vi "Read Active Channels.vi"(8 "error in (no error)":errorcluster, 11 "Hardware Settings in":refnum<class "Hardware Settings.lvclass">) -> (0 "error out":errorcluster, 2 "Active Channels":refnum<class "Generic Hardware.lvclass">[](array[class]), 3 "Hardware Settings out":refnum<class "Hardware Settings.lvclass">)   [LabVIEW 2017, in "Hardware Settings.lvclass"]
uses:
  Hardware Settings.lvclass
  Hardware Types/Generic/Generic Hardware.lvclass
  Hardware Settings.lvclass/Hardware Settings.ctl
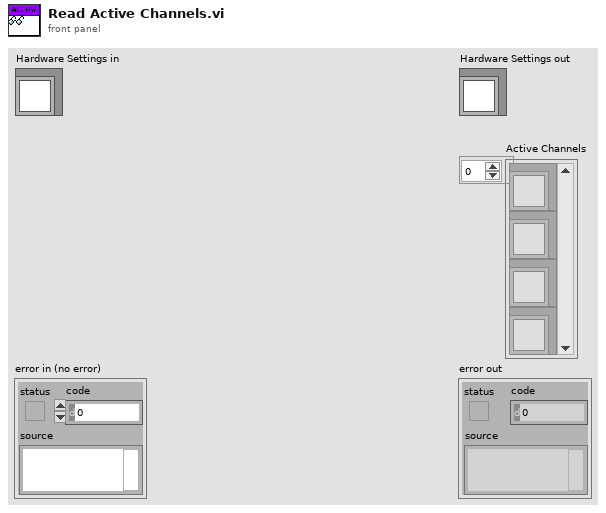
[diagram p1: front panel]
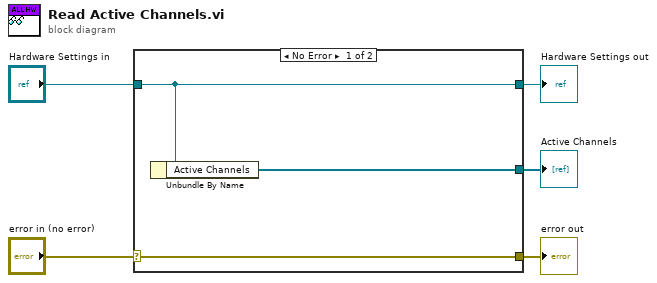
[diagram p0: block diagram]
diagram:
  n1 = case shown="No Error" "error in (no error)" {
    selector: "error in (no error)" -> [w8 w9]
    tunnel: [w8 w9] -> w4
    tunnel: [w7 w10] -> w2
    tunnel: "Hardware Settings in" -> [w7 w10]
    tunnel: [w6 _] -> w1
    frame No Error {
      n2 = Unbundle By Name(w7) -> ("Active Channels"=w6:refnum<class "Generic Hardware.lvclass">[])
    }
    frame Error {
    }
  }
  "error out" <- w4
  "Hardware Settings out" <- w2
  "Active Channels" <- w1
